vi "niRFUtil LCAPI Copy WFM (1 CSG).vi"(0 "Complex Waveform In":T1 {"y" format="%.2f"; "dx" format="%^.2e"; "x0" format="%^.2e"}, 11 "error in (no error)":errorcluster, 12 "Data Copy Descriptor":u64, 13 "Ignore Data Copy Descriptor":bool) -> (4 "Complex Waveform Out":T1 {"y" format="%.2f"; "dx" format="%^.2e"; "x0" format="%^.2e"}, 15 "error out":errorcluster)   [LabVIEW 2015, in "niRFUtil.lvlib"]
uses:
  niRFUtil.lvlib
  Includes/niRFUtil INC Complex Waveform.ctl
  Includes/niRFUtil INC Complex Array.ctl
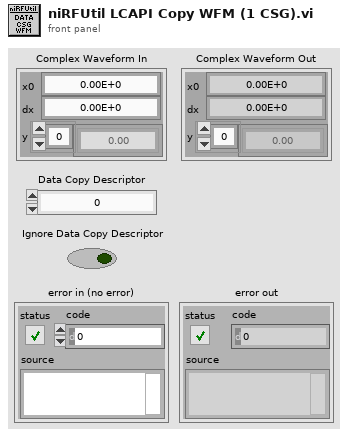
[diagram p1: front panel]
types:
  T1 = typedef "niRFUtil.lvlib/niRFUtil INC Complex Waveform.ctl" = cluster{"x0":dbl, "dx":dbl, "y":T2}
  T2 = typedef "niRFUtil.lvlib/niRFUtil INC Complex Array.ctl" = csg[]
  T3 = cluster{"status":bool, "return type":i32, "errorString":string}
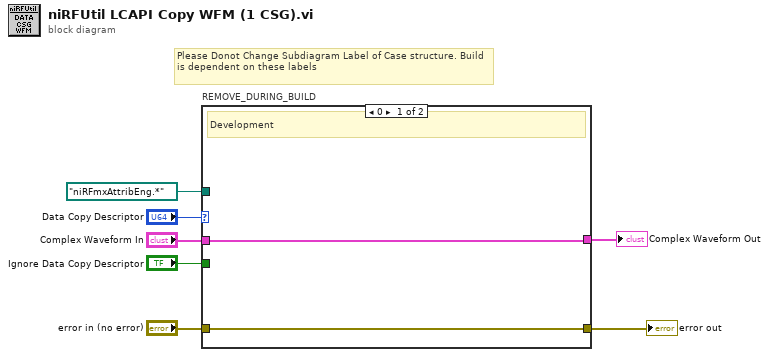
[diagram p0: block diagram]
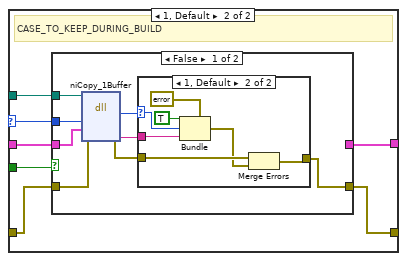
[diagram p2: hidden frame]
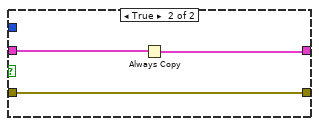
[diagram p4: hidden frame]
diagram:
  # "Please Donot Change Subdiagram Label of Case structure. Build is dependent on these labels"
  n1 = case "REMOVE_DURING_BUILD" shown="0" "Data Copy Descriptor" {
    selector: "Data Copy Descriptor" -> [_ w11]
    tunnel: "Complex Waveform In" -> [w8 w16]
    tunnel: [w9 w15] -> w6
    tunnel: "error in (no error)" -> [w9 w14]
    tunnel: [w8 w13] -> w4
    tunnel: "Ignore Data Copy Descriptor" -> [_ w12]
    tunnel: path "niRFmxAttribEng.*" ("path in") -> [_ w10]
    frame 0 {
      # "Development"
    }
    frame 1, Default {
      # "CASE_TO_KEEP_DURING_BUILD"
      n2 = case shown="False" w12 {
        tunnel: w14 -> [w24 w33]
        tunnel: w16 -> [w23 w34]
        tunnel: w11 -> [w22 _]
        tunnel: [w18 w33] -> w15
        tunnel: [_ w35] -> w13
        tunnel: w10 -> [w17 _]
        frame False {
          n3 = dll-call lib="niRFmxAttribEng.*" fn="niCopy_1Buffer"(path in=w17, error in=w24, "dataCopyDescriptor"=w22, "source"=w23) -> (error out=w19:errorcluster, "return type"=w20:i32, "errorString"=w21:string)  [unwired: 4 in, 1 out]
          n4 = case shown="1, Default" w20 {
            selector: w20 -> [_ w31]
            tunnel: w21 -> [_ w30]
            tunnel: w19 -> [w25 w28]
            tunnel: [w25 w29] -> w18
            frame 0 {
            }
            frame 1, Default {
              n5 = Bundle(cluster=T3 {"status"=FALSE, "return type"=0, "errorString"=""}, "status"=TRUE, "return type"=w31, "errorString"=w30) -> (w27:T3)
              n6 = Merge Errors(w28, w27) -> (w29:errorcluster)
            }
          }
        }
        frame True {
          n7 = Always Copy(1:w34) -> (0:w35:T1)
        }
      }
    }
  }
  "error out" <- w6
  "Complex Waveform Out" <- w4
